vi "create_line_messung.vi"(0 "B-Feld":dbl, 2 "Temperatur":dbl, 5 "Kapazität":dbl, 7 "Loss":dbl, 9 "Timestamp":dbl, 11 "Empty Line":bool) -> (10 "Ausgabe":string)   [LabVIEW 2009]
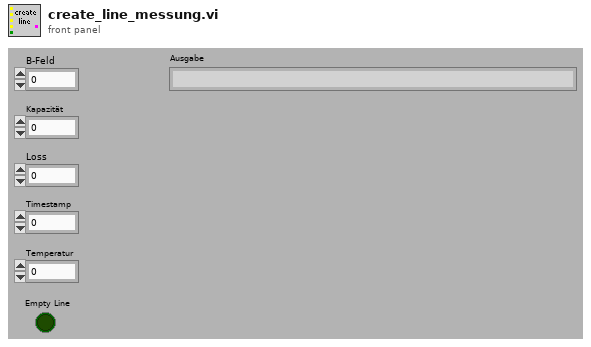
[diagram p1: front panel]
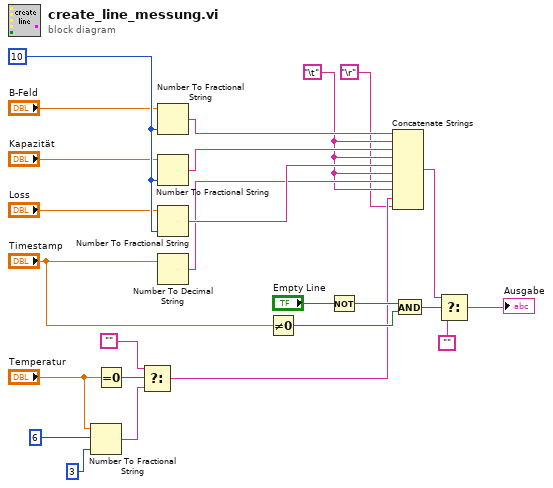
[diagram p0: block diagram]
diagram:
  w17 = "\t"
  w25 = 10
  n1 = Number To Fractional String(number="Temperatur", width (-)=6, precision (6)=3) -> (F-format string=w6:string)  [unwired: 1 in]
  n2 = Equal To 0?(x="Temperatur") -> (x = 0?=w8:bool)
  n3 = Select(t="", s=w8, f=w6) -> (s? t:f=w3:string)
  n4 = Number To Fractional String(number="B-Feld", precision (6)=w25) -> (F-format string=w21:string)  [unwired: 2 in]
  n5 = Number To Fractional String(number="Kapazität", precision (6)=w25) -> (F-format string=w20:string)  [unwired: 2 in]
  n6 = Number To Fractional String(number="Loss", precision (6)=w25) -> (F-format string=w19:string)  [unwired: 2 in]
  n7 = Number To Decimal String(number="Timestamp") -> (decimal integer string=w18:string)  [unwired: 1 in]
  n8 = Not Equal To 0?(x="Timestamp") -> (x != 0?=w9:bool)
  n9 = Not(x="Empty Line") -> (.not. x?=w10:bool)
  n10 = Concatenate Strings(w21, w17, w20, w17, w19, w17, w18, w17, w3, "\r") -> (w16:string)
  n11 = And(x=w10, y=w9) -> (x .and. y?=w11:bool)
  n12 = Select(t=w16, s=w11, f="") -> (s? t:f=→"Ausgabe":string)
